vi "FPGA Status String.vi"(8 "error in (no error)":errorcluster, 10 "Authorized":T1, 11 "Refnum in":T2) -> (0 "error out":errorcluster, 3 "Data String":string)   [LabVIEW 2020]
doc: "Author: Scott Hannahs <sth@magnet.fsu.edu>\nCopyright 2018 Florida State University, All rights reserved."
uses:
  RT Controls/FPGA SCH Digitizer Ref.ctl
  RT Controls/RT System Auth Level.ctl
  RT Controls/Status Info.ctl
  <vilib>/Utility/error.llb/Error Cluster From Error Code.vi
  <vilib>/rvi/errors/niLvFpgaAdjustHostInterfaceError.vi
  RT Host Globals.vi
  <vilib>/rvi/interface/nirviReadWriteControl/nirviReadWriteControl.xnode
  NiFpgaLv.dll
  <vilib>/rvi/interface/Simulation/niFpgaSimulationCallBeginRW.vi
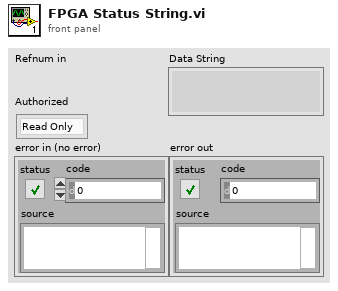
[diagram p1: front panel]
types:
  T1 = typedef "RT System Auth Level.ctl" = enum16{"Read Only", "Operator", "Admin"}
  T2 = typedef "FPGA SCH Digitizer Ref.ctl" = refnum<k20>
  T3 = typedef "Status Info.ctl" = cluster{"VT Error Array":bool[], "Joint Err Array":bool[], "SC Bus Err Array":bool[], "HTS Lead FRZ Err Array":bool[], "HTS Lead WarnErr Array":bool[], "HTS Bus Err Array":bool[], "RT Bus Err Array":bool[], "Resistive Status":cluster{"Bore Tube Fault":bool, "Coil V Faults":bool[], "Temp Faults":bool[], "Pressure Fault":bool, "Current Fault":bool, "Coil Volt Fault":bool, "I*Temp Fault":bool, "Dump File Enable":bool, "Active":bool}, "Pressure Limit Err Array":bool[], "DAQ Zero Fault Channel":bool[], "PS Enable First Error":u32, "Breaker First Error":u64, "Overall Errors":cluster{"RT Bus Limit Err":bool, "HTS Bus Limit Err":bool, "Pressure Limit Err":bool, "ResMag Limit Err":bool, "SC Bus Limit Err":bool, "Co-Wound Limit Err":bool, "Joint Limit Err":bool, "VT Quench Err":bool, "All Breaker Fault":bool, "Cooldown Mode":bool}, "Breaker Enable":bool, "PS Enable":bool, "Digitizer Read OK":bool, "Chassis Temperature":fxp<+/-,16,14>, "Pwr ±15V Pri Err":bool, "Pwr ±15V Aux Err":bool, "Pwr 5V Pri Err":bool, "Pwr 5V Aux Err":bool, "Pwr 24V Pri Err":bool, "Pwr 24V Aux Err":bool, "Pwr 125V Err":bool, "Breaker Pos 1 Closed":bool, "Breaker Pos 2 Closed":bool, "Breaker Pos 3 Closed":bool, "Breaker Neg 4 Closed":bool, "Breaker Neg 5 Closed":bool, "Breaker Neg 6 Closed":bool, "Low Current Mode":bool, "All Breakers Closed":bool, "Authorized":T1, "Reset Digitizers":bool, "Reset Breaker":bool, "Reset PS Enable":bool, "# Clients":u32}
  T4 = cluster{"RT Bus Limit Err":bool, "HTS Bus Limit Err":bool, "Pressure Limit Err":bool, "ResMag Limit Err":bool, "SC Bus Limit Err":bool, "Co-Wound Limit Err":bool, "Joint Limit Err":bool, "VT Quench Err":bool, "All Breaker Fault":bool, "Cooldown Mode":bool}
  T5 = cluster{"Bore Tube Fault":bool, "Coil V Faults":bool[], "Temp Faults":bool[], "Pressure Fault":bool, "Current Fault":bool, "Coil Volt Fault":bool, "I*Temp Fault":bool, "Dump File Enable":bool, "Active":bool}
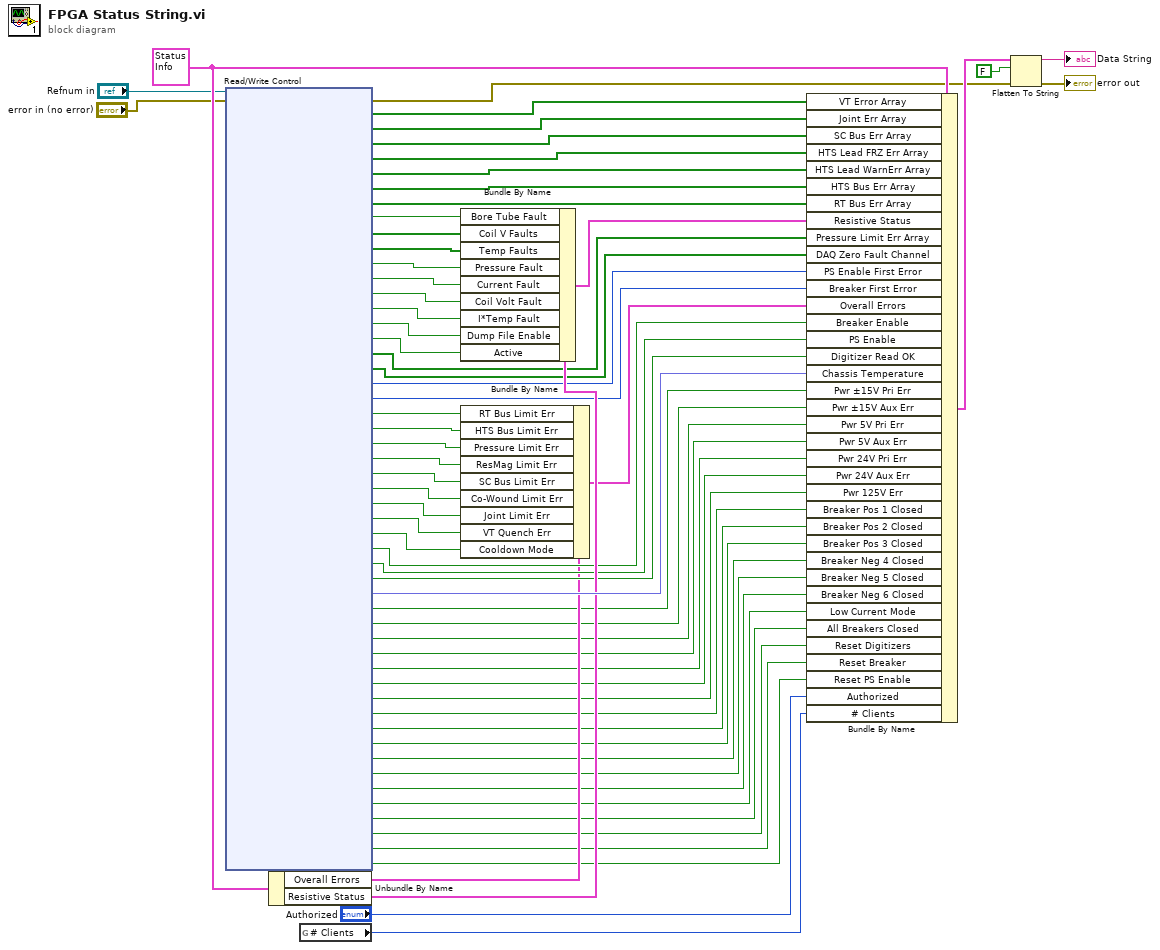
[diagram p0: block diagram]
diagram:
  w56 = T3 {"VT Error Array"=[FALSE, FALSE, FALSE, FALSE, FALSE, FALSE, FALSE, FALSE, FALSE, FALSE, FALSE, FALSE, FALSE, FALSE, FALSE, FALSE], "Joint Err Array"=[FALSE, FALSE, FALSE, FALSE, FALSE, FALSE, FALSE, FALSE], "SC Bus Err Array"=[FALSE, FALSE], "HTS Lead FRZ Err Array"=[FALSE, FALSE], "HTS Lead WarnErr Array"=[FALSE, FALSE], "HTS Bus Err Array"=[FALSE, FALSE], "RT Bus Err Array"=[FALSE, FALSE], "Resistive Status"={"Bore Tube Fault"=FALSE, "Coil V Faults"=[FALSE, FALSE, FALSE, FALSE], "Temp Faults"=[FALSE, FALSE, FALSE, FALSE], "Pressure Fault"=FALSE, "Current Fault"=FALSE, "Coil Volt Fault"=FALSE, "I*Temp Fault"=FALSE, "Dump File Enable"=FALSE, "Active"=FALSE}, "Pressure Limit Err Array"=[FALSE, FALSE, FALSE, FALSE], "DAQ Zero Fault Channel"=[FALSE, FALSE, FALSE, FALSE, FALSE, FALSE, FALSE, FALSE, FALSE, FALSE, FALSE, FALSE, FALSE, FALSE, FALSE, FALSE, FALSE, FALSE, FALSE, FALSE, FALSE, FALSE, FALSE, FALSE, FALSE, FALSE, FALSE, FALSE, FALSE, FALSE, FALSE, FALSE, FALSE, FALSE, FALSE, FALSE, FALSE, FALSE], "PS Enable First Error"=0, "Breaker First Error"=0, "Overall Errors"={"RT Bus Limit Err"=FALSE, "HTS Bus Limit Err"=FALSE, "Pressure Limit Err"=FALSE, "ResMag Limit Err"=FALSE, "SC Bus Limit Err"=FALSE, "Co-Wound Limit Err"=FALSE, "Joint Limit Err"=FALSE, "VT Quench Err"=FALSE, "All Breaker Fault"=FALSE, "Cooldown Mode"=FALSE}, "Breaker Enable"=FALSE, "PS Enable"=FALSE, "Digitizer Read OK"=FALSE, "Chassis Temperature"=0.0, "Pwr ±15V Pri Err"=FALSE, "Pwr ±15V Aux Err"=FALSE, "Pwr 5V Pri Err"=FALSE, "Pwr 5V Aux Err"=FALSE, "Pwr 24V Pri Err"=FALSE, "Pwr 24V Aux Err"=FALSE, "Pwr 125V Err"=FALSE, "Breaker Pos 1 Closed"=FALSE, "Breaker Pos 2 Closed"=FALSE, "Breaker Pos 3 Closed"=FALSE, "Breaker Neg 4 Closed"=FALSE, "Breaker Neg 5 Closed"=FALSE, "Breaker Neg 6 Closed"=FALSE, "Low Current Mode"=FALSE, "All Breakers Closed"=FALSE, "Authorized"=enum."Read Only", "Reset Digitizers"=FALSE, "Reset Breaker"=FALSE, "Reset PS Enable"=FALSE, "# Clients"=0} ("SCH Status")
  n1 = xnode "Read/Write Control"("FPGA VI Reference In"="Refnum in", "error in"="error in (no error)") -> ("error out"=w21:errorcluster, "VT Error Array"=w25:bool[], "Joint Err Array"=w26:bool[], "SC Bus Err Array"=w27:bool[], "HTS Lead FRZ Err Array"=w28:bool[], "HTS Lead Warn Err Array"=w29:bool[], "HTS Bus Err Array"=w30:bool[], "RT Bus Err Array"=w31:bool[], "Bore Tube Fault"=w60:bool, "Coil V Faults"=w33:bool[], "Temp Faults"=w34:bool[], "Pressure Fault"=w35:bool, "Current Fault"=w36:bool, "Coil Volt Fault"=w37:bool, "I*Temp Fault"=w38:bool, "Dump File Enable"=w39:bool, "Active"=w40:bool, "Pressure Limit Err Array"=w41:bool[], "DAQ Zero Fault Channel"=w42:bool[], "PS Enable First Error"=w43:u32, "Breaker First Error"=w44:u64, "RT Bus Limit Err"=w47:bool, "HTS Bus Limit Err"=w48:bool, "Pressure Limit Err"=w49:bool, "ResMag Limit Err"=w50:bool, "SC Bus Limit Err"=w51:bool, "Co-Wound Limit Err"=w52:bool, "Joint Limit Err"=w53:bool, "VT Quench Err"=w54:bool, "Cooldown Mode"=w1:bool, "Breaker Enable"=w57:bool, "PS Enable"=w58:bool, "Digitizer Read OK"=w59:bool, "Chassis Temperature"=w65:fxp<+/-,16,14>, "Pwr +/-15V Pri Err"=w23:bool, "Pwr +/-15V Aux Err"=w20:bool, "Pwr 5V Pri Err"=w19:bool, "Pwr 5V Aux Err"=w18:bool, "Pwr 24V Pri Err"=w17:bool, "Pwr 24V Aux Err"=w16:bool, "Pwr 125V Err"=w15:bool, "Breaker Pos 1 Closed"=w14:bool, "Breaker Pos 2 Closed"=w13:bool, "Breaker Pos 3 Closed"=w12:bool, "Breaker Neg 4 Closed"=w11:bool, "Breaker Neg 5 Closed"=w10:bool, "Breaker Neg 6 Closed"=w9:bool, "Low Current Mode"=w8:bool, "All Breakers Closed"=w7:bool, "Reset Digitizers"=w5:bool, "Reset Breaker"=w4:bool, "Reset PS Enable"=w3:bool)  [unwired: 1 out]
  n2 = Unbundle By Name(w56) -> ("Overall Errors"=w45:T4, "Resistive Status"=w64:T5)
  n3 = global read "RT Host Globals.vi" "# Clients"() -> (w2:u32)
  n4 = Bundle By Name(cluster=w64, "Bore Tube Fault"=w60, "Coil V Faults"=w33, "Temp Faults"=w34, "Pressure Fault"=w35, "Current Fault"=w36, "Coil Volt Fault"=w37, "I*Temp Fault"=w38, "Dump File Enable"=w39, "Active"=w40) -> (w32:T5)
  n5 = Bundle By Name(cluster=w45, "RT Bus Limit Err"=w47, "HTS Bus Limit Err"=w48, "Pressure Limit Err"=w49, "ResMag Limit Err"=w50, "SC Bus Limit Err"=w51, "Co-Wound Limit Err"=w52, "Joint Limit Err"=w53, "VT Quench Err"=w54, "Cooldown Mode"=w1) -> (w46:T4)
  n6 = Bundle By Name(cluster=w56, "VT Error Array"=w25, "Joint Err Array"=w26, "SC Bus Err Array"=w27, "HTS Lead FRZ Err Array"=w28, "HTS Lead WarnErr Array"=w29, "HTS Bus Err Array"=w30, "RT Bus Err Array"=w31, "Resistive Status"=w32, "Pressure Limit Err Array"=w41, "DAQ Zero Fault Channel"=w42, "PS Enable First Error"=w43, "Breaker First Error"=w44, "Overall Errors"=w46, "Breaker Enable"=w57, "PS Enable"=w58, "Digitizer Read OK"=w59, "Chassis Temperature"=w65, "Pwr ±15V Pri Err"=w23, "Pwr ±15V Aux Err"=w20, "Pwr 5V Pri Err"=w19, "Pwr 5V Aux Err"=w18, "Pwr 24V Pri Err"=w17, "Pwr 24V Aux Err"=w16, "Pwr 125V Err"=w15, "Breaker Pos 1 Closed"=w14, "Breaker Pos 2 Closed"=w13, "Breaker Pos 3 Closed"=w12, "Breaker Neg 4 Closed"=w11, "Breaker Neg 5 Closed"=w10, "Breaker Neg 6 Closed"=w9, "Low Current Mode"=w8, "All Breakers Closed"=w7, "Reset Digitizers"=w5, "Reset Breaker"=w4, "Reset PS Enable"=w3, "Authorized"="Authorized", "# Clients"=w2) -> (w61:T3)
  n7 = Flatten To String(anything=w61, prepend array or string size? (T)=FALSE, error in (no error)=w21) -> (data string=→"Data String":string, error out=→"error out":errorcluster)  [unwired: 1 in, 1 out]
